vi "Untitled 2 (SubVI).vi"(9 "c":dbl, 10 "b":dbl, 11 "a":dbl) -> (3 "x":dbl)   [LabVIEW 2016]
uses:
  <vilib>/express/express arith-compare/Formula/XNode/ExpressFormulaBlockNode.xnode
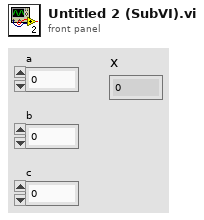
[diagram p1: front panel]
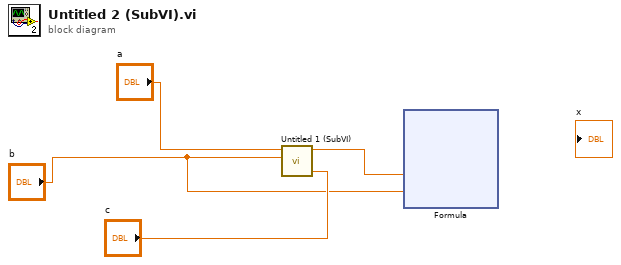
[diagram p0: block diagram]
diagram:
  n1 = call "Untitled 1 (SubVI).vi"("c"="c", "b"="b", "a"="a") -> ("D"=w2:dbl)  [unwired: 8 in]
  n2 = xnode "Formula"("D"=w2, "b"="b") -> ()  [unwired: 2 in, 2 out]
